vi "grab and display.vi"() -> ()   [LabVIEW 2013]
panel:
  out "ms between image":u32
  out "Frame Rate":dbl
  in  "Stop (F)":bool
  out "Image Out":T1(plugin-control)
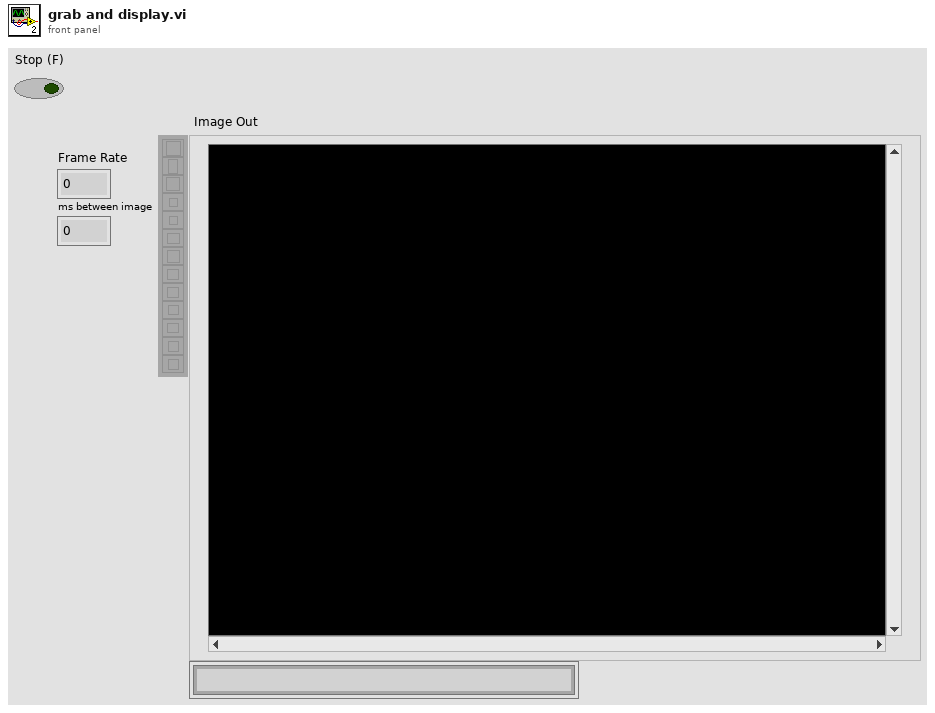
[diagram p1: front panel]
types:
  T1 = typedef "IMAQ Image.ctl" = refnum<image>
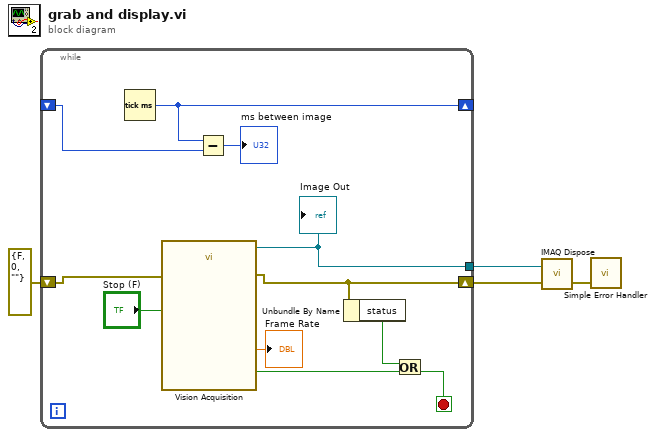
[diagram p0: block diagram]
diagram:
  n1 = while {
    shift-right: [w12] -> _
    shift-left: _ -> [w11]
    shift-right: [w7] -> w4
    shift-left: errorcluster {"status"=FALSE, "code"=0, "source"=""} ("error out") -> [w8]
    tunnel: [w5] -> w2
    stop <- w9 stop-if-true
    n2 = Tick Count (ms)() -> (millisecond timer value=w12:u32)
    n3 = call "Vision Acquisition"("Stop (F)"="Stop (F)", "error in"=w8) -> ("Image Out"=w5:T1, "Frame Rate"=→"Frame Rate":dbl, "Stopped"=w14:bool, "error out"=w7:errorcluster)  [unwired: 22 in]
    "Image Out" <- w5
    n4 = Subtract(x=w12, y=w11) -> (x-y=→"ms between image":u32)
    n5 = Unbundle By Name(w7) -> ("status"=w6:bool)
    n6 = Or(x=w6, y=w14) -> (x .or. y?=w9:bool)
  }
  n7 = call "IMAQ Dispose"("Image"=w2, "error in (no error)"=w4) -> ("error out"=w1:errorcluster)  [unwired: 4 in]
  n8 = call <vilib>:"Simple Error Handler.vi"("error in (no error)"=w1) -> ()  [unwired: 4 in, 5 out]
